vi "WriteLogFile.vi"(7 "Data File":string, 8 "Error In":errorcluster, 9 "DUT passed?":bool, 10 "Value TechSpec criteria":dbl, 11 "Files saved?":bool) -> (0 "Error Out":errorcluster)   [LabVIEW 2018]
uses:
  globals/QC_RunInformation.vi
panel:
  out "Cause for quitting measurement":string
  in  "OK Button":bool
  in  "Add comment":bool
  out "Type of measurement":string
  out "Logfile entry":string
  # "Write Logfile"
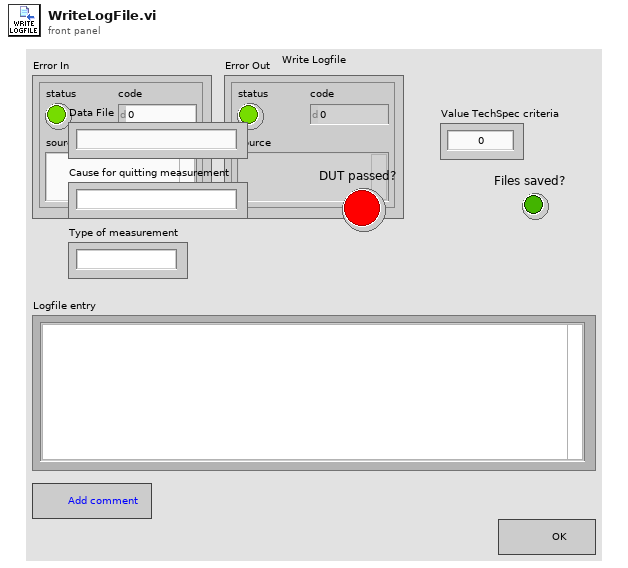
[diagram p1: front panel]
types:
  T1 = enum16{"open", "replace", "create", "open or create", "replace or create", "replace or create with confirmation"}
  T2 = cluster{"Sensor Serial No.:":string, "Wafer Serial No.:":string, "Batch:":string, "Manufacturer:":string, "Device Category:":string, "Database Serial No.:":string, "Initiated:":string, "Test":string, "Instruments used:":string, "Probeplan used:":string, "End of Run comment:":string, "User:":string}
  T3 = cluster{"Institute":string, "Manufacturers":string[], "Devices":string[], "Serialnumbers Lookup DB":string, "Data directory":string, "Backup & screenshot directory":string, "List of known users":string[]}
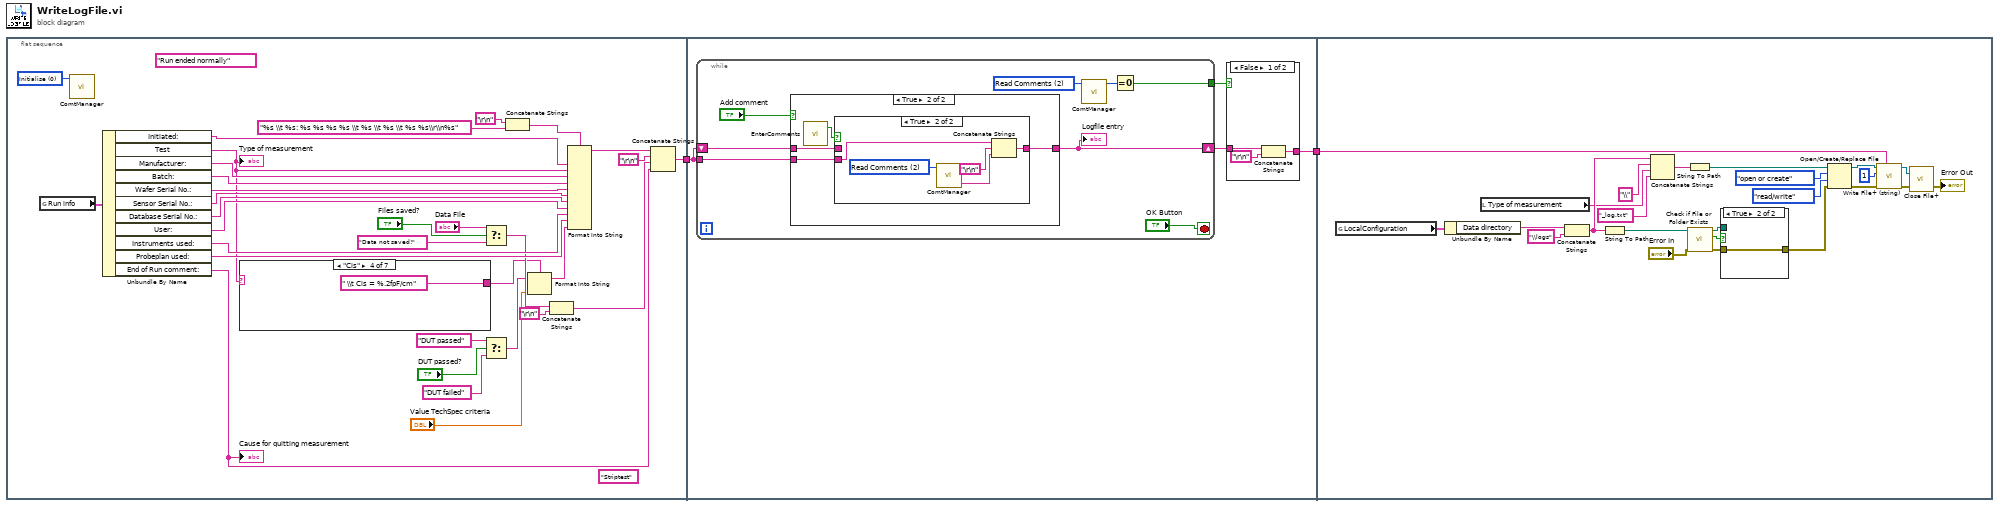
[diagram p0: block diagram]
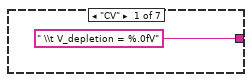
[diagram p2: hidden frame]
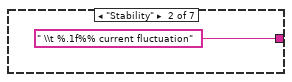
[diagram p3: hidden frame]
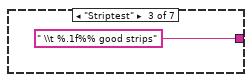
[diagram p4: hidden frame]
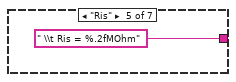
[diagram p5: hidden frame]
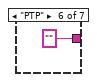
[diagram p6: hidden frame]
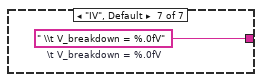
[diagram p7: hidden frame]
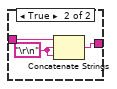
[diagram p8: hidden frame]
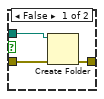
[diagram p11: hidden frame]
diagram:
  n1 = flat-sequence {
    tunnel: [w28] -> w2
    tunnel: w2 -> [w45]
    tunnel: [w43] -> w1
    tunnel: w1 -> [w86]
    frame #0 {
      (unwired) "Run ended normally" ("Cause for quitting measurement")
      (unwired) "Striptest"
      w27 = u16 0 items=["Initialise", "Add comment", "Read Comments"] ("Action")
      n2 = global read "QC_RunInformation.vi" "Run info"() -> (w26:T2)
      n3 = call "ComtManager.vi"("Action"=w27) -> ()  [unwired: 2 in, 3 out]
      n4 = Unbundle By Name(w26) -> ("Initiated:"=w34:string, "Test"=w6:string, "Manufacturer:"=w24:string, "Batch:"=w23:string, "Wafer Serial No.:"=w22:string, "Sensor Serial No.:"=w21:string, "Database Serial No.:"=w20:string, "User:"=w19:string, "Instruments used:"=w18:string, "Probeplan used:"=w17:string, "End of Run comment:"=w8:string)
      "Type of measurement" <- w6
      "Cause for quitting measurement" <- w8
      n5 = case shown="\"Cis\"" w6 {
        tunnel: [" \\t V_depletion = %.0fV" " \\t %.1f%% current fluctuation" " \\t %.1f%% good strips" " \\t Cis = %.2fpF/cm" " \\t Ris = %.2fMOhm" "" w41] -> w5
        frame "CV" {
        }
        frame "Stability" {
        }
        frame "Striptest" {
        }
        frame "Cis" {
        }
        frame "Ris" {
        }
        frame "PTP" {
        }
        frame "IV", Default {
          w41 = " \\t V_breakdown = %.0fV"  # \t V_breakdown = %.0fV
        }
      }
      n6 = Select(t="Data File", s="Files saved?", f="Data not saved!") -> (s? t:f=w10:string)
      n7 = Select(t="DUT passed", s="DUT passed?", f="DUT failed") -> (s? t:f=w4:string)
      n8 = Concatenate Strings("\r\n", "%s \\t %s: %s %s %s %s \\t %s \\t %s \\t %s %s\\r\\n%s") -> (w32:string)
      n9 = Format Into String(format string=w5, initial string=w4, "Value TechSpec criteria") -> (resulting string=w3:string)  [unwired: 1 in, 1 out]
      n10 = Concatenate Strings(w10, "\r\n") -> (w29:string)
      n11 = Format Into String(format string=w32, w34, w6, w24, w23, w22, w21, w20, w19, w18, w17, w3) -> (resulting string=w30:string)  [unwired: 2 in, 1 out]
      n12 = Concatenate Strings(w30, "\r\n", w29, w8) -> (w28:string)
    }
    frame #1 {
      n13 = while {
        shift-right: [w55] -> w44
        shift-left: w45 -> [w57]
        tunnel: w45 -> [w56]
        tunnel: [w52] -> w42
        stop <- "OK Button" stop-if-true
        w54 = u16 2 items=["Initialise", "Add comment", "Read Comments"] ("Action")
        n14 = case shown="True" "Add comment" {
          tunnel: [w60 w63] -> w55
          tunnel: w57 -> [w60 w62]
          tunnel: w56 -> [_ w61]
          frame False {
          }
          frame True {
            n15 = call "EnterComments.vi"() -> ("update?"=w64:bool)  [unwired: 4 in]
            n16 = case shown="True" w64 {
              tunnel: [w65 w69] -> w63
              tunnel: w62 -> [w65 _]
              tunnel: w61 -> [_ w68]
              frame False {
              }
              frame True {
                w70 = u16 2 items=["Initialise", "Add comment", "Read Comments"] ("Action")
                n17 = call "ComtManager.vi"("Action"=w70) -> ("Comment out"=w67:string)  [unwired: 2 in, 2 out]
                n18 = Concatenate Strings(w68, "\r\n", w67) -> (w69:string)
              }
            }
          }
        }
        "Logfile entry" <- w55
        n19 = call "ComtManager.vi"("Action"=w54) -> ("No of comments"=w53:i32)  [unwired: 2 in, 2 out]
        n20 = Equal To 0?(x=w53) -> (x = 0?=w52:bool)
      }
      n21 = case shown="False" w42 {
        tunnel: w44 -> [w47 w49]
        tunnel: [w46 w50] -> w43
        frame False {
          n22 = Concatenate Strings(w47, "\r\n") -> (w46:string)
        }
        frame True {
          w51 = "\r\n"
          n23 = Concatenate Strings(w49, w51, w51) -> (w50:string)
        }
      }
    }
    frame #2 {
      n24 = global read "QC_RunInformation.vi" "LocalConfiguration"() -> (w85:T3)
      n25 = Unbundle By Name(w85) -> ("Data directory"=w83:string)
      n26 = local read "Type of measurement"() -> (w71:string)
      n27 = Concatenate Strings(w83, "\\logs") -> (w80:string)
      n28 = String To Path(string=w80) -> (path=w77:path)
      n29 = Concatenate Strings(w80, "\\", w71, "_log.txt") -> (w79:string)
      n30 = String To Path(string=w79) -> (path=w78:path)
      n31 = call <vilib>:"Check if File or Folder Exists.vi"("error in (no error)"="Error In", "path"=w77) -> ("error out"=w73:errorcluster, "file or folder exists?"=w76:bool, "dup path"=w75:path)  [unwired: 7 in]
      n32 = case shown="True" w76 {
        tunnel: w75 -> [w97 _]
        tunnel: w73 -> [w96 w98]
        tunnel: [w95 w98] -> w72
        frame False {
          n33 = Create Folder(path (use dialog)=w97, error in=w96) -> (error out=w95:errorcluster)  [unwired: 1 in, 2 out]
        }
        frame True {
        }
      }
      n34 = Open/Create/Replace File(file path (use dialog)=w78, error in=w72, operation (0:open)=T1."open or create", access (0:read/write)=enum16{"read/write", "read-only", "write-only"}."read/write") -> (refnum out=w91:refnum<file>, error out=w92:errorcluster)  [unwired: 2 in, 1 out]
      n35 = call <vilib>:"Write File+ (string).vi"("string"=w86, "error in (no error)"=w92, "pos mode (rel. to end:1)"=1, "refnum"=w91) -> ("error out"=w88:errorcluster, "dup refnum"=w87:refnum<file>)  [unwired: 3 in, 1 out]
      n36 = call <vilib>:"Close File+.vi"("error in (no error)"=w88, "refnum"=w87) -> ("error out"=→"Error Out":errorcluster)  [unwired: 3 in, 2 out]
    }
  }
